vi "RegTester.vi"() -> ()   [LabVIEW 2012]
uses:
  <vilib>/vision/NI_Vision_Development_Module.lvlib
  <vilib>/Utility/file.llb/Write To Spreadsheet File (DBL).vi
  Registration method.ctl
panel:
  out "Image":T1(plugin-control)
  in  "Registration method":T2
  out "alignment quality":dbl[](graph)
  out "x translation":dbl[](graph)
  in  "x translation file":path
  in  "quality array file":path
  out "error out":errorcluster
  in  "Registration parameters":T3={"Sampling Percentage"=0.2, "maximum iteration"=200, "number of bins"=200}
  in  "image folder":path
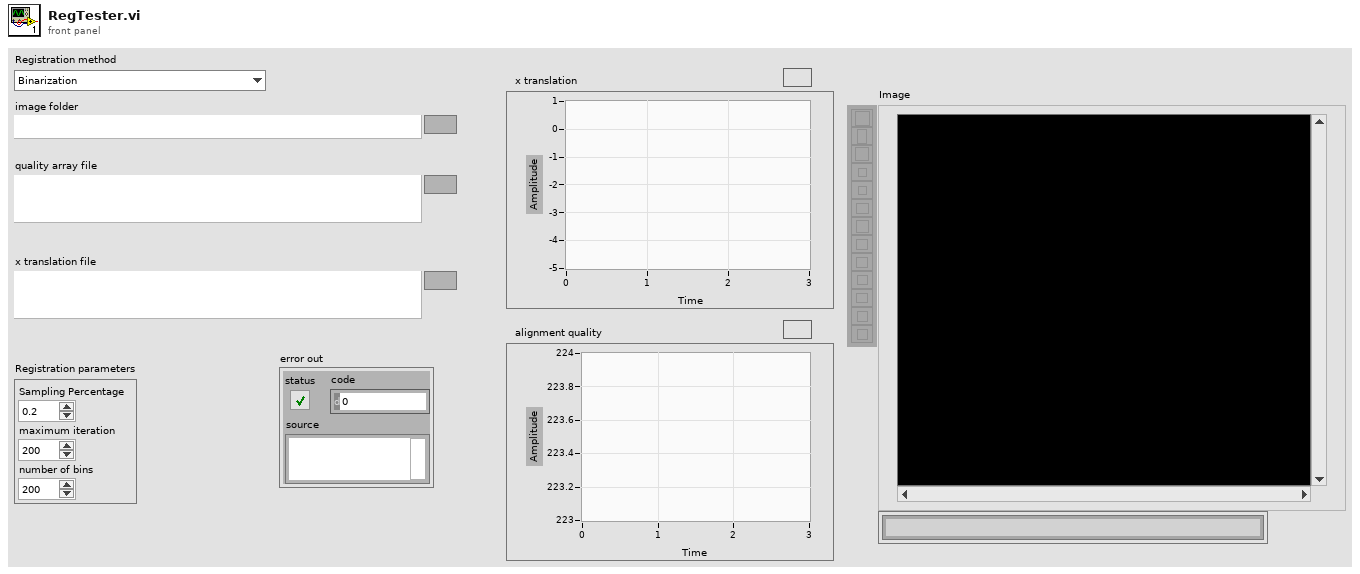
[diagram p1: front panel]
types:
  T1 = typedef "IMAQ Image.ctl" = refnum<image>
  T2 = typedef "Registration method.ctl" = enum16{"Binarization", "Difference of Gaussians", "Edges Detection", "Gaussians and Binarization", "Edges and Gaussians", "Edges and Binarization", "All"}
  T3 = cluster{"Sampling Percentage":dbl, "maximum iteration":i32, "number of bins":u32}
  T4 = typedef "Image Type" = u32
  T5 = typedef "ROI Descriptor" = cluster{"Global Rectangle":i32[], "Contours":cluster{"ID":enum32{"External", "Internal"}, "Type":u32, "Coordinates":i32[]}[]}
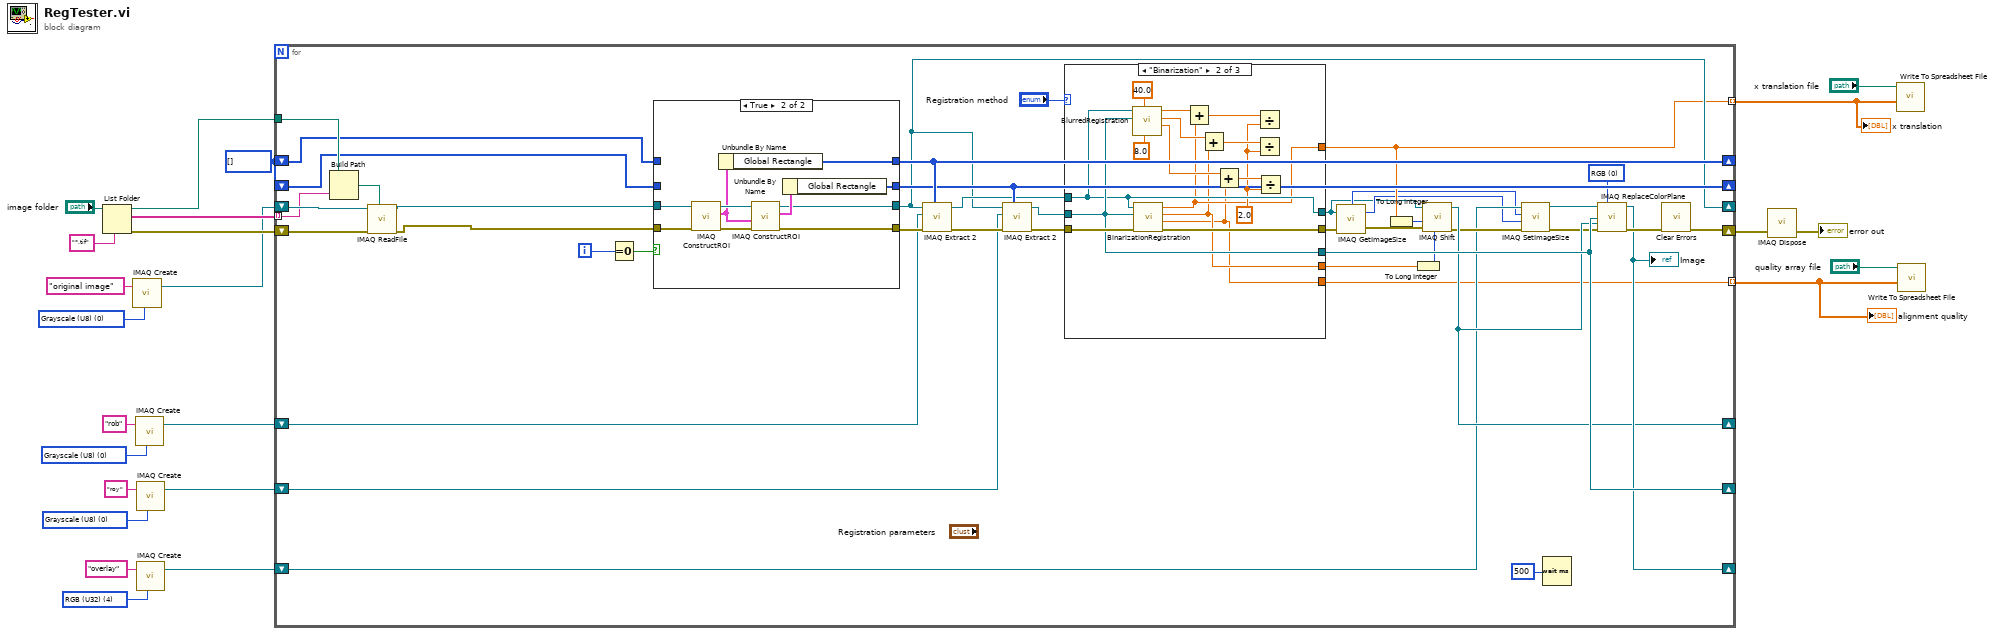
[diagram p0: block diagram]
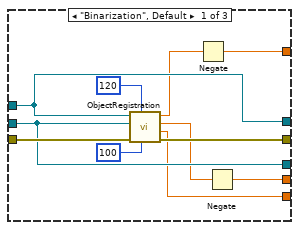
[diagram p2: hidden frame]
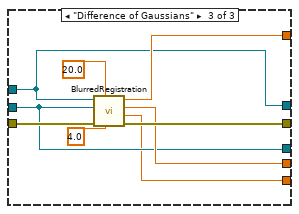
[diagram p3: hidden frame]
diagram:
  w10 = i32[] [] ("Global Rectangle")
  w13 = T4 4 items=["Grayscale (U8)", "Grayscale (I16)", "Grayscale (SGL)", "Complex (CSG)", "RGB (U32)", "HSL (U32)", "RGB (U64)", "Grayscale (U16)"] ("Image Type")
  w15 = T4 0 items=["Grayscale (U8)", "Grayscale (I16)", "Grayscale (SGL)", "Complex (CSG)", "RGB (U32)", "HSL (U32)", "RGB (U64)", "Grayscale (U16)"] ("Image Type")
  w16 = T4 0 items=["Grayscale (U8)", "Grayscale (I16)", "Grayscale (SGL)", "Complex (CSG)", "RGB (U32)", "HSL (U32)", "RGB (U64)", "Grayscale (U16)"] ("Image Type")
  w17 = T4 0 items=["Grayscale (U8)", "Grayscale (I16)", "Grayscale (SGL)", "Complex (CSG)", "RGB (U32)", "HSL (U32)", "RGB (U64)", "Grayscale (U16)"] ("Image Type")
  n1 = List Folder(path="image folder", pattern="*.tif") -> (path out=w11:path, filenames=w19:string[], error out=w18:errorcluster)  [unwired: 2 in, 1 out]
  n2 = call "IMAQ Create"("Image Name"="original image", "Image Type"=w17) -> ("New Image"=w12:T1)  [unwired: 3 in, 1 out]
  n3 = call "IMAQ Create"("Image Name"="rob", "Image Type"=w16) -> ("New Image"=w9:T1)  [unwired: 3 in, 1 out]
  n4 = call "IMAQ Create"("Image Name"="roy", "Image Type"=w15) -> ("New Image"=w8:T1)  [unwired: 3 in, 1 out]
  n5 = call "IMAQ Create"("Image Name"="overlay", "Image Type"=w13) -> ("New Image"=w7:T1)  [unwired: 3 in, 1 out]
  n6 = for {
    tunnel: w19 -> [w64] mode=indexing
    shift-right: [w50] -> w3
    shift-left: w18 -> [w67]
    shift-right: [w47] -> _
    shift-left: w12 -> [w66]
    tunnel: w11 -> [w65]
    shift-right: [w56] -> _
    shift-left: w10 -> [w59]
    shift-right: [w53] -> _
    shift-left: w10 -> [w60]
    shift-right: [w40] -> _
    shift-left: w9 -> [w57]
    shift-right: [w46] -> _
    shift-left: w8 -> [w54]
    shift-right: [w42] -> _
    shift-left: w7 -> [w37]
    tunnel: [w44] -> w4 mode=indexing
    tunnel: [w29] -> w1 mode=indexing
    i -> [w62]
    w41 = u16 0 items=["RGB", "HSL", "HSV", "HSI"] ("Color Mode")
    n7 = Build Path(base path=w65, name or relative path=w64) -> (appended path=w63:path)
    n8 = call "IMAQ ReadFile"("File Path"=w63, "error in (no error)"=w67, "Image"=w66) -> ("error out"=w27:errorcluster, "Image Out"=w26:T1)  [unwired: 4 in, 3 out]
    n9 = Equal To 0?(x=w62) -> (x = 0?=w61:bool)
    n10 = case shown="True" w61 {
      tunnel: w27 -> [w105 w117]
      tunnel: w26 -> [w106 w116]
      tunnel: [w105 w111] -> w58
      tunnel: [w106 w110] -> w47
      tunnel: [w107 w109] -> w53
      tunnel: [w104 w108] -> w56
      tunnel: w60 -> [w107 _]
      tunnel: w59 -> [w104 _]
      frame False {
      }
      frame True {
        n11 = call "IMAQ ConstructROI"("error in (no error)"=w117, "Image"=w116) -> ("error out"=w114:errorcluster, "ROI Descriptor Out"=w113:T5, "Image Out (duplicate)"=w115:T1)  [unwired: 6 in, 1 out]
        n12 = Unbundle By Name(w113) -> ("Global Rectangle"=w108:i32[])
        n13 = call "IMAQ ConstructROI"("error in (no error)"=w114, "ROI Descriptor In (None)"=w113, "Image"=w115) -> ("error out"=w111:errorcluster, "ROI Descriptor Out"=w112:T5, "Image Out (duplicate)"=w110:T1)  [unwired: 5 in, 1 out]
        n14 = Unbundle By Name(w112) -> ("Global Rectangle"=w109:i32[])
      }
    }
    n15 = call "IMAQ Extract 2"("Optional Rectangle"=w56, "error in (no error)"=w58, "Image Dst"=w57, "Image Src"=w47) -> ("error out"=w55:errorcluster, "Image Dst Out"=w51:T1)  [unwired: 6 in]
    n16 = call "IMAQ Extract 2"("Optional Rectangle"=w53, "error in (no error)"=w55, "Image Dst"=w54, "Image Src"=w47) -> ("error out"=w52:errorcluster, "Image Dst Out"=w25:T1)  [unwired: 6 in]
    n17 = case shown="\"Binarization\"" "Registration method" {
      tunnel: w52 -> [w78 w94 w103]
      tunnel: w51 -> [w76 w91 w97]
      tunnel: w25 -> [w75 w92 w96]
      tunnel: [w77 w93 w102] -> w34
      tunnel: [w71 w81 w99] -> w44
      tunnel: [w70 w80 w98] -> w30
      tunnel: [w76 w91 w97] -> w31
      tunnel: [w75 w92 w96] -> w46
      tunnel: [w72 w79 w95] -> w29
      frame "Binarization", Default {
        n18 = call "ObjectRegistration.vi"("Min Size"=100, "Threshold"=120, "error in (no error)"=w78, "Roy"=w75, "Rob"=w76) -> ("error out"=w77:errorcluster, "Alignment quality"=w72:dbl, "y displacement"=w73:dbl, "x displacement"=w74:dbl)  [unwired: 3 in]
        n19 = Negate(x=w74) -> (-x=w71:dbl)
        n20 = Negate(x=w73) -> (-x=w70:dbl)
      }
      frame "Binarization" {
        w82 = 2.0 ("y")
        n21 = call "BlurredRegistration.vi"(6:sgl 8.0 ("small sigma"), 7:sgl 40.0 ("large sigma"), "roy"=w92, "rob"=w91) -> ("alignment quality"=w86:dbl, "y displacement"=w87:dbl, "x displacement"=w88:dbl)  [unwired: 4 in, 1 out]
        n22 = call "BinarizationRegistration.vi"("error in"=w94, "Roy"=w92, "Rob"=w91) -> ("error out"=w93:errorcluster, "quality"=w79:dbl, "y translation"=w80:dbl, "x translation"=w81:dbl)  [unwired: 5 in]
        n23 = Add(x=w88, y=w81) -> (x+y=w85:dbl)
        n24 = Add(x=w87, y=w80) -> (x+y=w83:dbl)
        n25 = Add(x=w86, y=w79) -> (x+y=w84:dbl)
        n26 = Divide(x=w85, y=w82) -> ()  [unwired: 1 out]
        n27 = Divide(x=w83, y=w82) -> ()  [unwired: 1 out]
        n28 = Divide(x=w84, y=w82) -> ()  [unwired: 1 out]
      }
      frame "Difference of Gaussians" {
        n29 = call "BlurredRegistration.vi"(6:sgl 4.0 ("small sigma"), 7:sgl 20.0 ("large sigma"), "error in"=w103, "roy"=w96, "rob"=w97) -> ("error out"=w102:errorcluster, "alignment quality"=w95:dbl, "y displacement"=w98:dbl, "x displacement"=w99:dbl)  [unwired: 3 in]
      }
    }
    n30 = call "IMAQ GetImageSize"("Image"=w31, "error in (no error)"=w34) -> ("Y Resolution"=w32:i32, "X Resolution"=w33:i32, "error out"=w35:errorcluster)  [unwired: 2 in]
    n31 = To Long Integer(number=w44) -> (32bit integer=w45:i32)
    n32 = To Long Integer(number=w30) -> (32bit integer=w43:i32)
    n33 = call "IMAQ Shift"("YOffset"=w43, "error in (no error)"=w35, "XOffset"=w45, "Image Src"=w31) -> ("error out"=w39:errorcluster, "Image Dst Out"=w40:T1)  [unwired: 6 in]
    n34 = call "IMAQ SetImageSize"("error in (no error)"=w39, "Y Resolution"=w32, "X Resolution"=w33, "Image"=w37) -> ("error out"=w38:errorcluster, "Image Out"=w36:T1)  [unwired: 1 in]
    n35 = Wait (ms)(milliseconds to wait=u32 500) -> ()  [unwired: 1 out]
    n36 = call "IMAQ ReplaceColorPlane"("Image Src"=w36, "Color Mode"=w41, "Red or Hue Plane"=w46, "Green or Sat Plane"=w40, "error in (no error)"=w38) -> ("Image Dst Out"=w42:T1, "error out"=w48:errorcluster)  [unwired: 9 in]
    "Image" <- w42
    n37 = call <vilib>:"Clear Errors.vi"("error in (no error)"=w48) -> ("error out"=w50:errorcluster)  [unwired: 6 in]
  }
  "x translation" <- w4
  "alignment quality" <- w1
  n38 = call "IMAQ Dispose"("error in (no error)"=w3) -> ("error out"=→"error out":errorcluster)  [unwired: 5 in]
  n39 = call-poly <vilib>:"Write To Spreadsheet File.vi"("1D data"=w4, "file path (dialog if empty)"="x translation file") -> ()  [unwired: 6 in, 1 out]
  n40 = call-poly <vilib>:"Write To Spreadsheet File.vi"("1D data"=w1, "file path (dialog if empty)"="quality array file") -> ()  [unwired: 6 in, 1 out]
